vi "Main.vi"   [LabVIEW 2020]
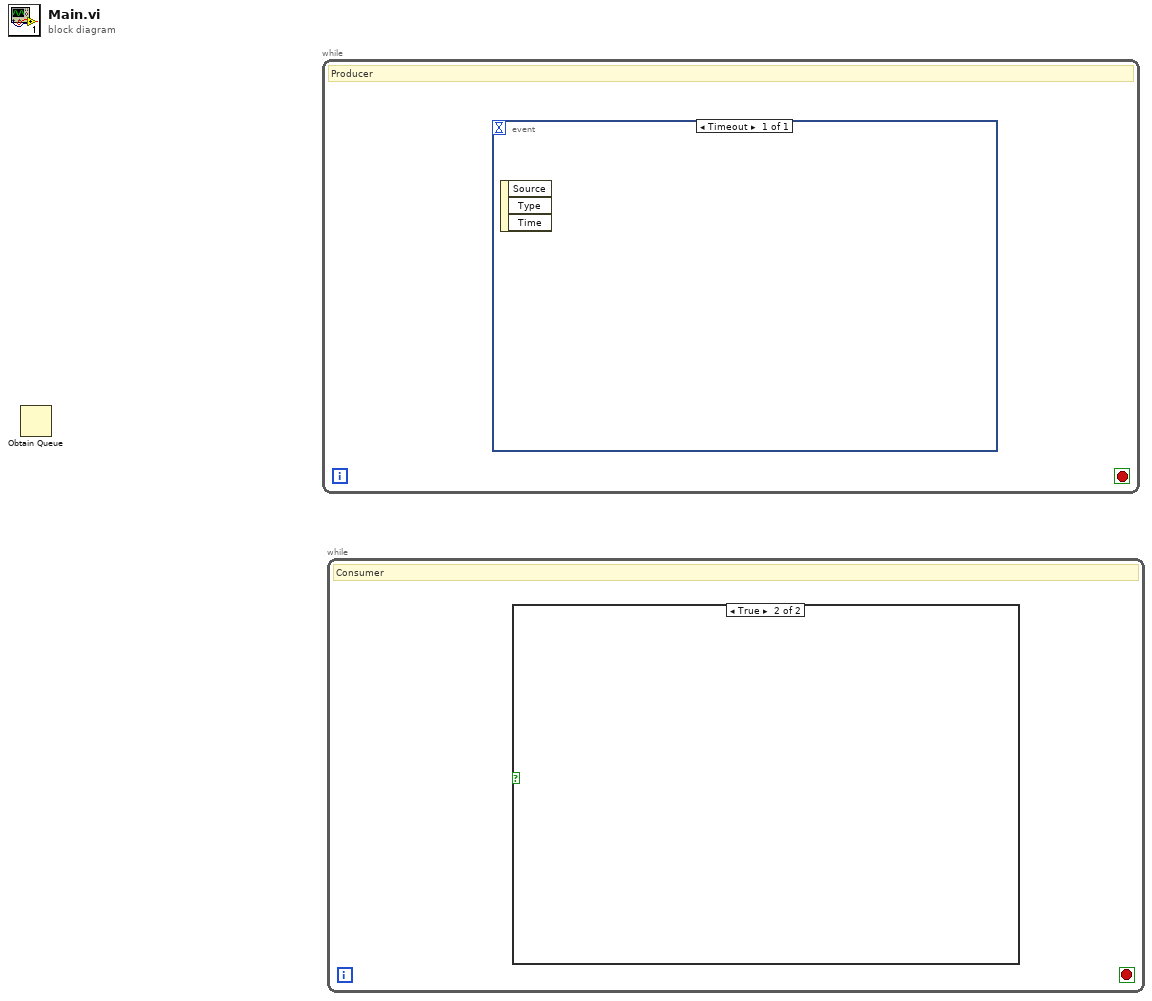
[diagram p0: block diagram]
diagram:
  n1 = Obtain Queue() -> ()  [unwired: 5 in, 3 out]
  n2 = while {
    stop <- _ stop-if-true
    # "Producer"
    n3 = event shown="[0] Timeout" {
      selector: _ -> [_]
      dyn-events: _ -> [_]
      timeout: _ -> [_]
      event Timeout {
        n4 = event-data() -> ()  [unwired: 1 in, 3 out]
      }
    }
  }
  n5 = while {
    stop <- _ stop-if-true
    # "Consumer"
    n6 = case shown="True" {
      selector: _ -> [_ _]
      frame False {
      }
      frame True {
      }
    }
  }
